vi "CS_cRIO-PB_DP-Master_SlaveIOData.vi"(0 "FPGA VI Reference":T1, 5 "Slave":i8, 7 "Modify output data":u8[](array[numeric]) format="%.0x", 11 "Error":errorcluster) -> (4 "FPGA VI Reference out":T1, 6 "Input data":u8[](array[numeric]) format="%.0x", 8 "Output data":u8[](array[numeric]) format="%.0x", 10 "Slave status":u8 format="%.0x", 12 "Output length":u8, 14 "Input length":u8, 15 "Error out":errorcluster)   [LabVIEW 2013, in "dynamic profibus.lvlib"]
doc: "Handles the cyclic process data of the selected DP-Slave.\n\nFPGA VI Reference:\nReference of the FPGA VI.\n\nSlave:\nPROFIBUS address of the DP-Slave. \n\nModify output data:\nThe Modify output data array contains the DP-Slave output data to be changed.\n\nInput data:\nThe Input data array contains the DP-Slave input data.\n\nOutput data:\nThe Output data array contains the DP-Slave output data.\n\nInput length:\nReturns the configured input length of the DP-Slave.\n\nOutput length:\nReturns the configured output length of the DP-Slave.\n\nSlave status:\n0x00: DP-Slave is in DataExchange mode, input and output data are valid\n0xC3: DP-Slave is not in Data Exchange mode, input and output data are invalid, DP-Slave diagnostic data are reported in Diag data array\n0xFF: DP-Slave is in Data Exchange mode and reports ext. diagnostic data, input and output data are valid.\n\nFPGA VI Reference out:\nIs a copy of the FPGA VI Reference .\n\nError in:\nPreceding error conditions. If an error has already occurred, the VI returns the value of the error in Error out.\n\nError out:\nError: TRUE if an error occurred.\nStatus: Error code\nInfo: Error description"
uses:
  dynamic profibus.lvlib
  fpga reference.ctl
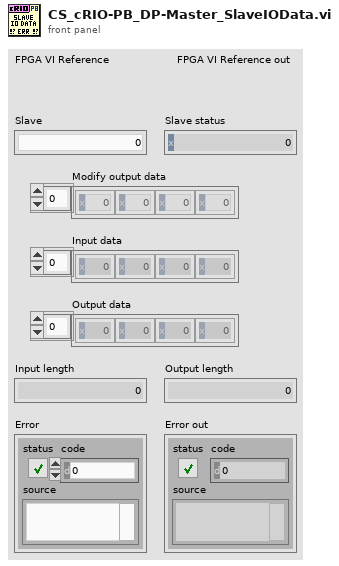
[diagram p1: front panel]
types:
  T1 = typedef "dynamic profibus.lvlib/fpga reference.ctl" = refnum<k20>
  T2 = enum16{"Start/Stop DP-Master", "Get Input Data", "Set Output Data", "Get Output Data", "Get Diagnostic Data", "Read/Write Data", "Read Diagnostic Data", "Get DPV1 Data", "Set DPV1 Data", "Read/Write DPV1 Data"}
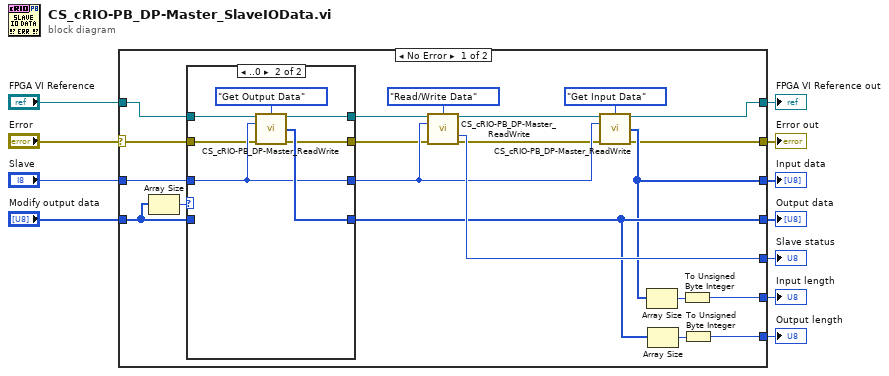
[diagram p0: block diagram]
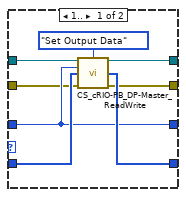
[diagram p2: hidden frame]
diagram:
  n1 = case shown="No Error" "Error" {
    selector: "Error" -> [w26 w48]
    tunnel: "Slave" -> [w28 _]
    tunnel: "FPGA VI Reference" -> [w27 w49]
    tunnel: "Modify output data" -> [w23 _]
    tunnel: [w30 _] -> w7
    tunnel: [w18 w49] -> w6
    tunnel: [w21 w48] -> w5
    tunnel: [w32 _] -> w4
    tunnel: [w31 _] -> w3
    tunnel: [w14 _] -> w2
    tunnel: [w16 _] -> w1
    frame No Error {
      n2 = Array Size(array=w23) -> (size(s)=w22:i32)
      n3 = case shown="..0" w22 {
        tunnel: w23 -> [w37 _]
        tunnel: w28 -> [w36 w44]
        tunnel: w27 -> [w35 w43]
        tunnel: w26 -> [w34 w42]
        tunnel: [w39 w46] -> w25
        tunnel: [w38 w45] -> w24
        tunnel: [w40 w47] -> w31
        tunnel: [w36 w44] -> w29
        frame 1.. {
          n4 = call "CS_cRIO-PB_DP-Master_ReadWrite.vi"("FPGA VI Reference"=w35, "Mode"=T2."Set Output Data", "Slave"=w36, "Data"=w37, "Error"=w34) -> ("FPGA VI Reference out"=w38:T1, "Data out"=w40:u8[], "Error out"=w39:errorcluster)  [unwired: 7 in, 1 out]
        }
        frame ..0 {
          n5 = call "CS_cRIO-PB_DP-Master_ReadWrite.vi"("FPGA VI Reference"=w43, "Mode"=T2."Get Output Data", "Slave"=w44, "Error"=w42) -> ("FPGA VI Reference out"=w45:T1, "Data out"=w47:u8[], "Error out"=w46:errorcluster)  [unwired: 8 in, 1 out]
        }
      }
      n6 = call "CS_cRIO-PB_DP-Master_ReadWrite.vi"("FPGA VI Reference"=w24, "Mode"=T2."Read/Write Data", "Slave"=w29, "Error"=w25) -> ("FPGA VI Reference out"=w19:T1, "Status"=w32:u8, "Error out"=w20:errorcluster)  [unwired: 8 in, 1 out]
      n7 = call "CS_cRIO-PB_DP-Master_ReadWrite.vi"("FPGA VI Reference"=w19, "Mode"=T2."Get Input Data", "Slave"=w29, "Error"=w20) -> ("FPGA VI Reference out"=w18:T1, "Data out"=w30:u8[], "Error out"=w21:errorcluster)  [unwired: 8 in, 1 out]
      n8 = Array Size(array=w30) -> (size(s)=w17:i32)
      n9 = Array Size(array=w31) -> (size(s)=w15:i32)
      n10 = To Unsigned Byte Integer(number=w17) -> (unsigned 8bit integer=w16:u8)
      n11 = To Unsigned Byte Integer(number=w15) -> (unsigned 8bit integer=w14:u8)
    }
    frame Error {
    }
  }
  "FPGA VI Reference out" <- w6
  "Input data" <- w7
  "Error out" <- w5
  "Slave status" <- w4
  "Output data" <- w3
  "Input length" <- w1
  "Output length" <- w2
